vi "CommandLineUploadWizardInt.vi"(4 "Arduino Base Path":path=path "C:/Program Files (x86)/Arduino", 5 "Progress Bar":refnum<vi>, 6 "Firmware Base Path":path, 7 "Upload COM Port":refnum<visa-resource-name>="N/A", 8 "Error In":errorcluster, 9 "Firmware Version":u16, 10 "Device Type":u16, 11 "Device Family":u8) -> (0 "Error Out":errorcluster, 3 "Log Path":path)   [LabVIEW 2019, in "LMH-LINX.lvlib"]
uses:
  <vilib>/MakerHub/LINX/LMH-LINX.lvlib
  <vilib>/MakerHub/Toolbox/LMH-Toolbox.lvlib
panel:
  out "Status":string
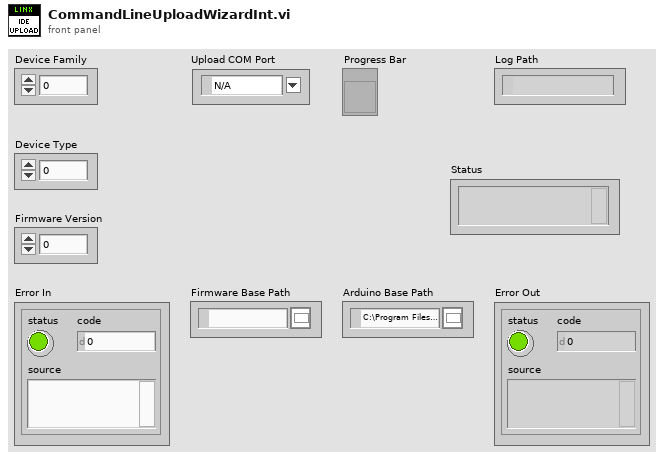
[diagram p1: front panel]
types:
  T1 = typedef "LVDateTimeRec.ctl" = cluster{"fractional second":dbl, "second":i32, "minute":i32, "hour":i32, "day of month":i32, "month":i32, "year":i32, "day of week":i32, "day of year":i32, "DST":i32}
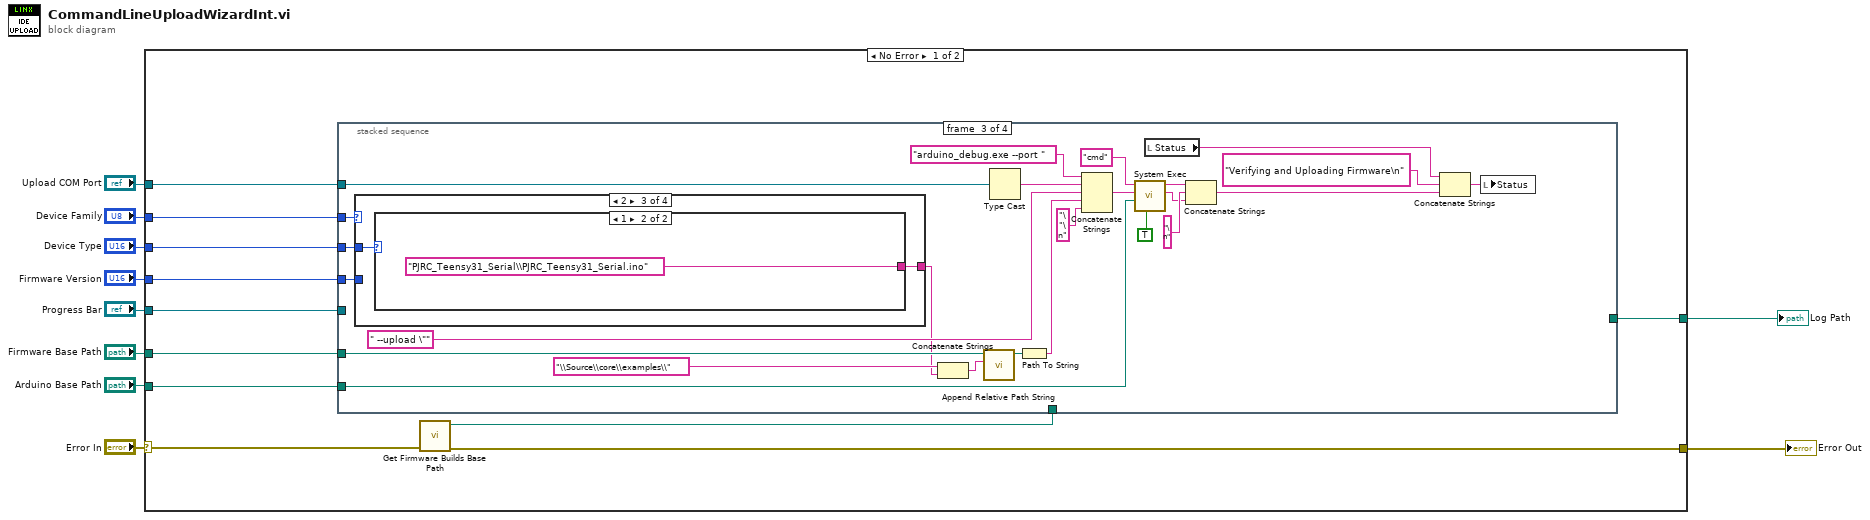
[diagram p0: block diagram]
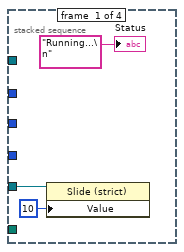
[diagram p2: hidden frame]
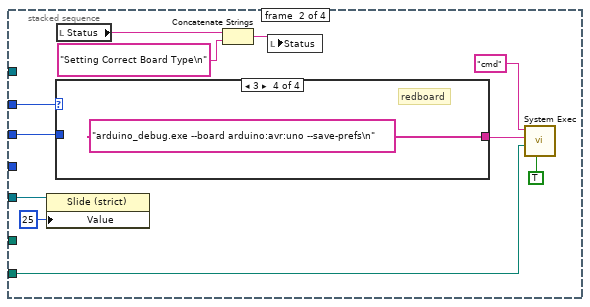
[diagram p3: hidden frame]
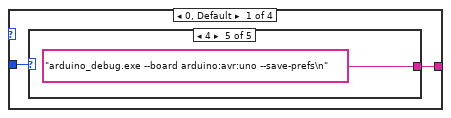
[diagram p4: hidden frame]
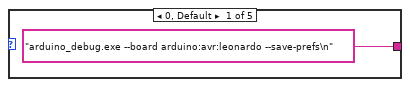
[diagram p5: hidden frame]
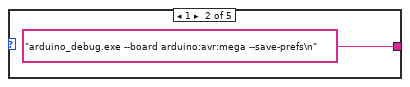
[diagram p6: hidden frame]
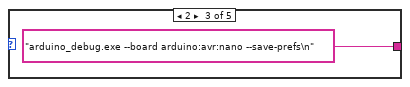
[diagram p7: hidden frame]
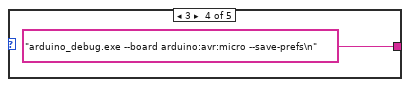
[diagram p8: hidden frame]
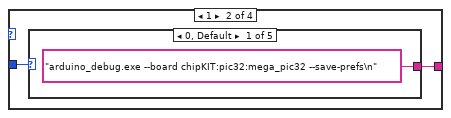
[diagram p9: hidden frame]
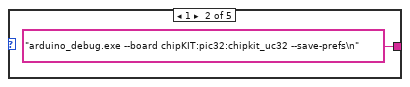
[diagram p10: hidden frame]
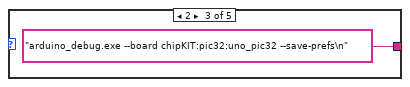
[diagram p11: hidden frame]
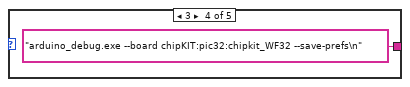
[diagram p12: hidden frame]
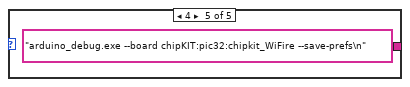
[diagram p13: hidden frame]
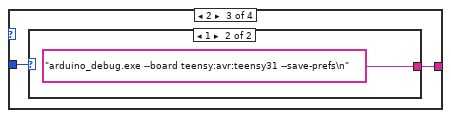
[diagram p14: hidden frame]
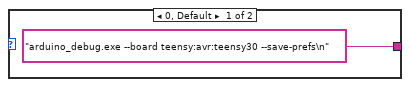
[diagram p15: hidden frame]
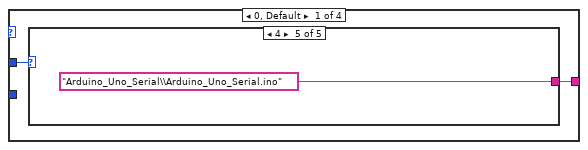
[diagram p16: hidden frame]
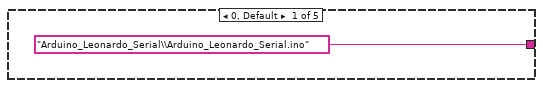
[diagram p17: hidden frame]
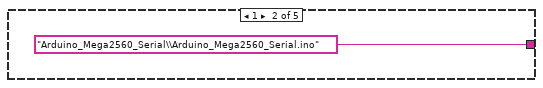
[diagram p18: hidden frame]
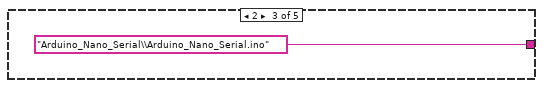
[diagram p19: hidden frame]
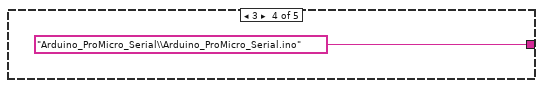
[diagram p20: hidden frame]
diagram:
  n1 = case shown="No Error" "Error In" {
    selector: "Error In" -> [w18 w140]
    tunnel: [w21 w140] -> w10
    tunnel: [w19 path ""] -> w9
    tunnel: "Arduino Base Path" -> [w17 _]
    tunnel: "Firmware Base Path" -> [w16 _]
    tunnel: "Progress Bar" -> [w15 _]
    tunnel: "Firmware Version" -> [w14 _]
    tunnel: "Device Type" -> [w13 _]
    tunnel: "Device Family" -> [w12 _]
    tunnel: "Upload COM Port" -> [w11 _]
    frame No Error {
      n2 = call <vilib>:"Get Firmware Builds Base Path.vi"("Error In"=w18) -> ("Error Out"=w21:errorcluster, "Firmware Builds Base Path"=w20:path)  [unwired: 9 in]
      n3 = stacked-sequence {
        tunnel: w11 -> [_ _ w71 _]
        tunnel: w12 -> [_ w33 w70 _]
        tunnel: w13 -> [_ w32 w69 _]
        tunnel: w14 -> [_ _ w68 _]
        tunnel: w15 -> [w24 w30 _ w137]
        tunnel: w16 -> [_ _ w63 _]
        tunnel: w17 -> [_ w25 w66 _]
        tunnel: w20 -> [_ _ _ w113]
        tunnel: [_ _ _ w111] -> w19
        frame #0 {
          n4 = property class="Slide (strict)"(reference=w24, "Value"=u8 10) -> ()  [unwired: 1 in, 2 out]
          "Status" <- "Running...\n" ("command line")
        }
        frame #1 {
          n5 = property class="Slide (strict)"(reference=w30, "Value"=u8 25) -> ()  [unwired: 1 in, 2 out]
          n6 = case shown="3" w33 {
            tunnel: w32 -> [w37 w44 w50 _]
            tunnel: [w36 w43 w51 "arduino_debug.exe --board arduino:avr:uno --save-prefs\n"] -> w31
            frame 0, Default {
              n7 = case shown="4" w37 {
                tunnel: ["arduino_debug.exe --board arduino:avr:leonardo --save-prefs\n" ("standard input") "arduino_debug.exe --board arduino:avr:mega --save-prefs\n" ("standard input") "arduino_debug.exe --board arduino:avr:nano --save-prefs\n" ("standard input") "arduino_debug.exe --board arduino:avr:micro --save-prefs\n" ("standard input") "arduino_debug.exe --board arduino:avr:uno --save-prefs\n" ("standard input")] -> w36
                frame 0, Default {
                }
                frame 1 {
                }
                frame 2 {
                }
                frame 3 {
                }
                frame 4 {
                }
              }
            }
            frame 1 {
              n8 = case shown="0, Default" w44 {
                tunnel: ["arduino_debug.exe --board chipKIT:pic32:mega_pic32 --save-prefs\n" ("standard input") "arduino_debug.exe --board chipKIT:pic32:chipkit_uc32 --save-prefs\n" ("standard input") "arduino_debug.exe --board chipKIT:pic32:uno_pic32 --save-prefs\n" ("standard input") "arduino_debug.exe --board chipKIT:pic32:chipkit_WF32 --save-prefs\n" ("standard input") "arduino_debug.exe --board chipKIT:pic32:chipkit_WiFire --save-prefs\n" ("standard input")] -> w43
                frame 0, Default {
                }
                frame 1 {
                }
                frame 2 {
                }
                frame 3 {
                }
                frame 4 {
                }
              }
            }
            frame 2 {
              n9 = case shown="1" w50 {
                tunnel: ["arduino_debug.exe --board teensy:avr:teensy30 --save-prefs\n" ("standard input") "arduino_debug.exe --board teensy:avr:teensy31 --save-prefs\n" ("standard input")] -> w51
                frame 0, Default {
                }
                frame 1 {
                }
              }
            }
            frame 3 {
              # "redboard"
            }
          }
          n10 = local read "Status"() -> (w28:string)
          n11 = Concatenate Strings(w28, "Setting Correct Board Type\n") -> (w26:string)
          n12 = local write "Status"(w26) -> ()
          n13 = call <vilib>:"System Exec.vi"("run minimized? (F)"=TRUE, "working directory"=w25, "standard input"=w31, "command line"="cmd") -> ()  [unwired: 4 in, 4 out]
        }
        frame #2 {
          n14 = case shown="2" w70 {
            tunnel: w69 -> [w81 w89 w106 _]
            tunnel: [w80 w88 w107 "Sparkfun_RedBoard_Serial\\Sparkfun_RedBoard_Serial.ino"] -> w61
            tunnel: w68 -> [_ w87 _ _]
            frame 0, Default {
              n15 = case shown="4" w81 {
                tunnel: ["Arduino_Leonardo_Serial\\Arduino_Leonardo_Serial.ino" "Arduino_Mega2560_Serial\\Arduino_Mega2560_Serial.ino" "Arduino_Nano_Serial\\Arduino_Nano_Serial.ino" "Arduino_ProMicro_Serial\\Arduino_ProMicro_Serial.ino" "Arduino_Uno_Serial\\Arduino_Uno_Serial.ino"] -> w80
                frame 0, Default {
                }
                frame 1 {
                }
                frame 2 {
                }
                frame 3 {
                }
                frame 4 {
                }
              }
            }
            frame 1 {
              n16 = case shown="1" w89 {
                tunnel: [w90 "ChipKIT_uC32_Serial\\ChipKIT_uC32_Serial.pde\"" "ChipKIT_Uno32_Serial\\ChipKIT_Uno32_Serial.pde\"" w97 w102] -> w88
                tunnel: w87 -> [w91 _ _ w96 w101]
                frame 0, Default {
                  n17 = case shown="0, Default" w91 {
                    tunnel: ["ChipKIT_Max32_Ethernet_Configurable\\ChipKIT_Max32_Ethernet_Configurable.pde\"" "ChipKIT_Max32_Serial\\ChipKIT_Max32_Serial.pde\""] -> w90
                    frame 0, Default {
                    }
                    frame 1 {
                    }
                  }
                }
                frame 1 {
                }
                frame 2 {
                }
                frame 3 {
                  n18 = case shown="0, Default" w96 {
                    tunnel: ["ChipKIT_WF32_Serial\\ChipKIT_WF32_Serial.pde\"" "ChipKIT_WF32_Wifi_Configurable\\ChipKIT_WF32_Wifi_Configurable.pde\"" "ChipKIT_WF32_Wifi_Configurable\\ChipKIT_WF32_Wifi_Configurable.pde\""] -> w97
                    frame 0, Default {
                    }
                    frame 1 {
                    }
                    frame 2 {
                    }
                  }
                }
                frame 4 {
                  n19 = case shown="0, Default" w101 {
                    tunnel: ["ChipKIT_WiFire_Serial\\ChipKIT_WiFire_Serial.pde\"" "ChipKIT_WiFire_Wifi_Configurable\\ChipKIT_WiFire_Wifi_Configurable.pde\"" "ChipKIT_WiFire_Wifi_Configurable\\ChipKIT_WiFire_Wifi_Configurable.pde\""] -> w102
                    frame 0, Default {
                    }
                    frame 1 {
                    }
                    frame 2 {
                    }
                  }
                }
              }
            }
            frame 2 {
              n20 = case shown="1" w106 {
                tunnel: ["PJRC_Teensy30_Serial\\PJRC_Teensy30_Serial.ino" "PJRC_Teensy31_Serial\\PJRC_Teensy31_Serial.ino"] -> w107
                frame 0, Default {
                }
                frame 1 {
                }
              }
            }
            frame 3 {
            }
          }
          n21 = Concatenate Strings("\\Source\\core\\examples\\" ("Relative Path"), w61) -> (w64:string)
          n22 = call <vilib>:"Append Relative Path String.vi"("Relative Path"=w64, "Base Path"=w63) -> ("Absolute Path"=w60:path)  [unwired: 8 in, 1 out]
          n23 = Type Cast(x=w71) -> (*(type *) &x=w76:string)  [unwired: 1 in]
          n24 = Path To String(path=w60) -> (string=w59:string)
          n25 = Concatenate Strings("arduino_debug.exe --port " ("Input"), w76, " --upload \"", w59, "\"\n" ("string")) -> (w78:string)
          n26 = call <vilib>:"System Exec.vi"("run minimized? (F)"=TRUE, "working directory"=w66, "standard input"=w78, "command line"="cmd") -> ("standard error"=w72:string, "standard output"=w74:string)  [unwired: 4 in, 2 out]
          n27 = local read "Status"() -> (w57:string)
          n28 = Concatenate Strings(w74, "\n", w72) -> (w55:string)
          n29 = Concatenate Strings(w57, "Verifying and Uploading Firmware\n" ("Status"), w55) -> (w56:string)
          n30 = local write "Status"(w56) -> ()
        }
        frame #3 {
          w134 = "_" ("string")
          w130 = i16 2 ("width (-)")
          n31 = local read "Status"() -> (w136:string)
          n32 = property class="Slide (strict)"(reference=w137, "Value"=u8 100) -> ()  [unwired: 1 in, 2 out]
          n33 = Concatenate Strings(w136, "\nDone" ("Status 2")) -> (w112:string)
          n34 = Get Date/Time In Seconds() -> (seconds since 1Jan1904=w117:timestamp)
          n35 = Seconds To Date/Time(time stamp (now)=w117) -> (date time rec=w116:T1)  [unwired: 1 in]
          n36 = Unbundle By Name(w116) -> ("year"=w118:i32, "month"=w119:i32, "day of month"=w120:i32, "hour"=w121:i32, "minute"=w122:i32, "second"=w131:i32)
          n37 = Number To Decimal String(number=w131, width (-)=w130) -> (decimal integer string=w133:string)
          n38 = Number To Decimal String(number=w119, width (-)=w130) -> (decimal integer string=w125:string)
          n39 = Number To Decimal String(number=w120, width (-)=w130) -> (decimal integer string=w126:string)
          n40 = Number To Decimal String(number=w121, width (-)=w130) -> (decimal integer string=w127:string)
          n41 = Number To Decimal String(number=w122, width (-)=w130) -> (decimal integer string=w128:string)
          n42 = Number To Decimal String(number=w118, width (-)=i16 4) -> (decimal integer string=w124:string)
          n43 = Concatenate Strings(w124, w134, w125, w134, w126, w134, w127, w134, w128, w134, w133, ".txt" ("string")) -> (w129:string)
          n44 = Build Path(base path=w113, name or relative path="Logs") -> (appended path=w115:path)
          n45 = Build Path(base path=w115, name or relative path=w129) -> (appended path=w111:path)
          n46 = Write to Text File(file (use dialog)=w111, text=w112) -> ()  [unwired: 2 in, 3 out]
        }
      }
    }
    frame Error {
    }
  }
  "Error Out" <- w10
  "Log Path" <- w9
